vi "RYB_labview_ardunio.vi"() -> ()   [LabVIEW 2013]
uses:
  D:/Program Files (x86)/National Instruments/LabVIEW 2013/examples/Instrument IO/Serial/support/Serial - Settings.ctl
  <vilib>/Instr/_visa.llb/VISA Configure Serial Port (Instr).vi
panel:
  out "B":dbl
  out "Y":dbl
  out "R":dbl
  in  "Boolean 5":bool
  out "B PHASE":bool
  out "Y PHASE":bool
  out "R PHASE":bool
  in  "stop":bool
  out "Input Data":i32(graph)
  out "FSR1":string
  out "Input buffer":string
  in  "byte count":u32
  in  "Serial Settings":T1={"baud rate"=9600, "data bits"=8, "parity"=enum."None", "stop bits"=10, "flow control"=0} {"flow control" items=["None"=0, "XON/XOFF"=1, "RTS/CTS"=2, "DTR/DSR"=4]; "stop bits" items=["1.0"=10, "1.5"=15, "2.0"=20]; "data bits" min=5 max=8 step=1; "baud rate" items=["75"=75, "110"=110, "134"=134, "150"=150, "300"=300, "600"=600, "1200"=1200, "1800"=1800, "2400"=2400, "4800"=4800, "7200"=7200, "9600"=9600, "14400"=14400, "19200"=19200, "28800"=28800, "38400"=38400, "56000"=56000, "57600"=57600, "115200"=115200, "128000"=128000, "230400"=230400]}
  in  "VISA resource name":refnum<visa-resource-name>
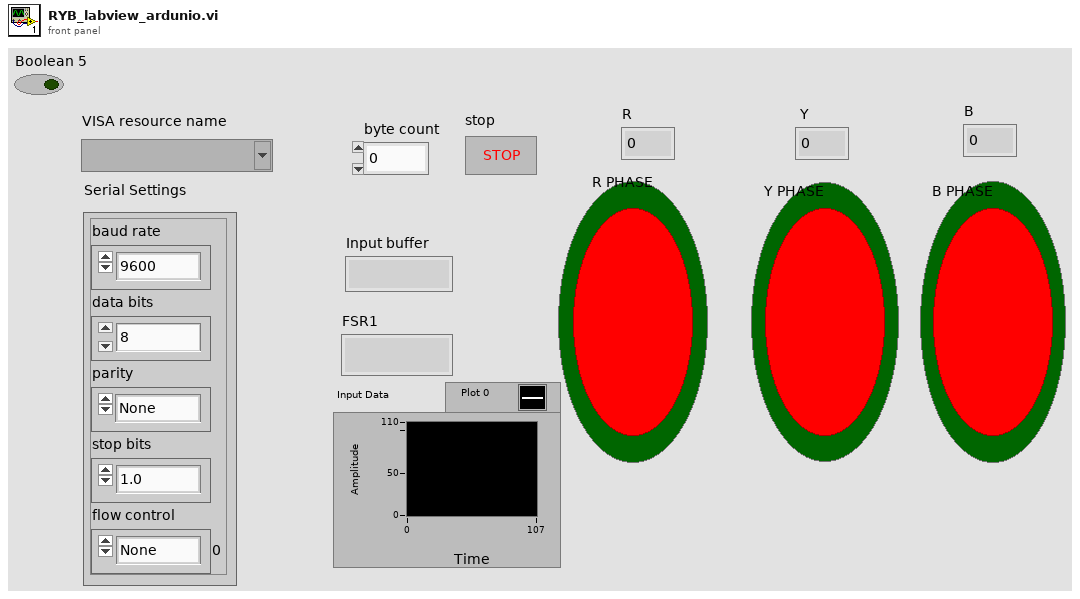
[diagram p1: front panel]
types:
  T1 = typedef "Serial - Settings.ctl" = cluster{"baud rate":u32, "data bits":u16, "parity":enum16{"None", "Odd", "Even", "Mark", "Space"}, "stop bits":u16, "flow control":u16}
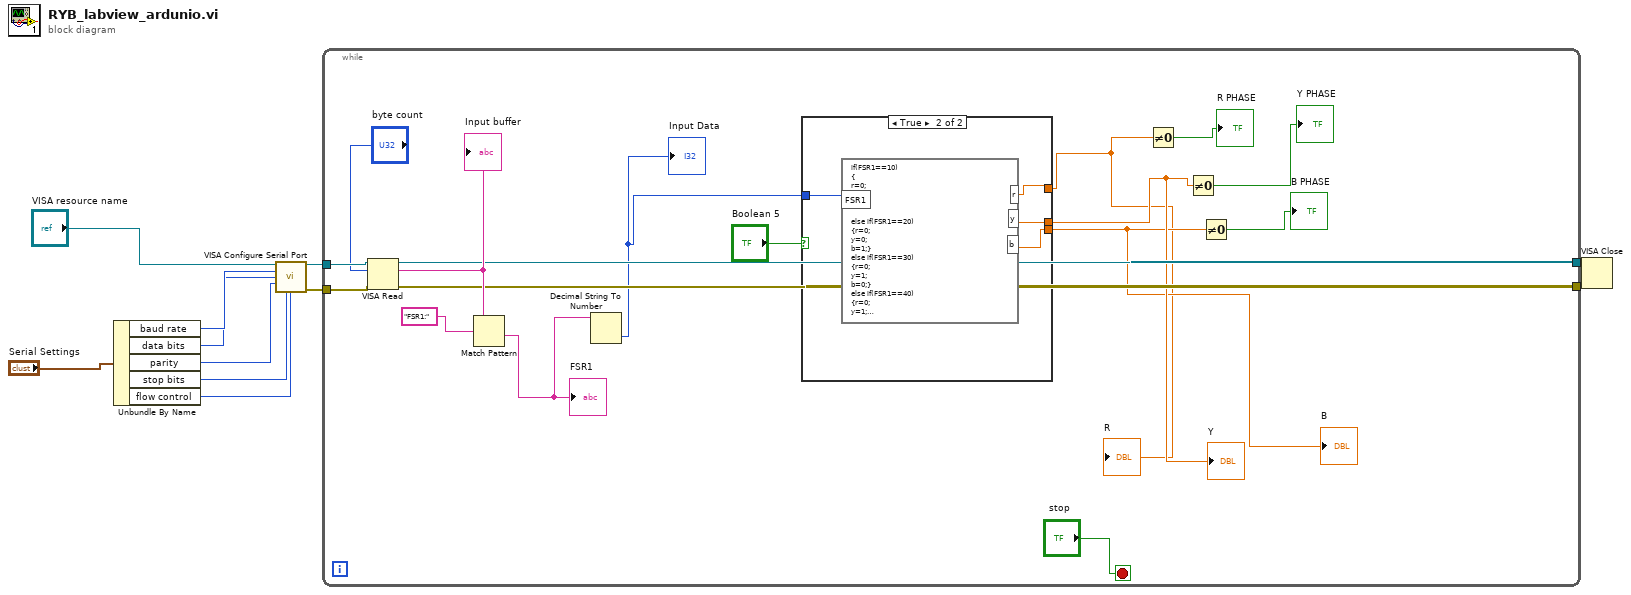
[diagram p0: block diagram]
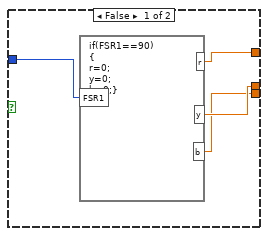
[diagram p2: hidden frame]
diagram:
  n1 = Unbundle By Name("Serial Settings") -> ("baud rate"=w9:u32, "data bits"=w8:u16, "parity"=w7:enum16{"None", "Odd", "Even", "Mark", "Space"}, "stop bits"=w6:u16, "flow control"=w5:u16)
  n2 = call-poly "VISA Configure Serial Port"("VISA resource name"="VISA resource name", "baud rate (9600)"=w9, "data bits (8)"=w8, "parity (0:none)"=w7, "stop bits (10: 1 bit)"=w6, "flow control (0:none)"=w5) -> ("VISA resource name out"=w4:refnum<visa-resource-name>, "error out"=w3:errorcluster)  [unwired: 8 in]
  n3 = while {
    tunnel: w4 -> [w28]
    tunnel: w3 -> [w27]
    tunnel: [w23] -> w2
    tunnel: [w22] -> w1
    stop <- "stop" stop-if-true
    n4 = VISA Read(VISA resource name=w28, byte count="byte count", error in (no error)=w27) -> (VISA resource name out=w22:refnum<visa-resource-name>, read buffer=w25:string, error out=w23:errorcluster)  [unwired: 1 out]
    "Input buffer" <- w25
    n5 = Match Pattern(string=w25, regular expression="FSR1:") -> (after substring=w20:string)  [unwired: 1 in, 3 out]
    "FSR1" <- w20
    n6 = Decimal String To Number(string=w20) -> (number=w17:i32)  [unwired: 2 in, 1 out]
    "Input Data" <- w17
    n7 = case shown="True" "Boolean 5" {
      tunnel: w17 -> [w32 w36]
      tunnel: [w30 w35] -> w15
      tunnel: [w29 w34] -> w14
      tunnel: [w31 w33] -> w12
      frame False {
        n8 = formula code="if(FSR1==90)\n{\nr=0;\ny=0;\nb=0;}"("FSR1"=w32) -> ("r"=w31:dbl, "y"=w30:dbl, "b"=w29:dbl)
      }
      frame True {
        n9 = formula code="if(FSR1==10)\n{\nr=0;\ny=0;\nb=0;}\n\nelse if(FSR1==20)\n{r=0;\ny=0;\nb=1;}\nelse if(FSR1==30)\n{r=0;\ny=1;\nb=0;}\nelse if(FSR1==40)\n{r=0;\ny=1;\nb=1;}\nelse if(FSR1==50)\n{r=1;\ny=0;\nb=0;}\nelse if(FSR1==60)\n{r=1;\ny=0;\nb=1;}\nelse if(FSR1==70)\n{r=1;\ny=1;\nb=0;}\nelse if(FSR1==80)\n{r=1;\ny=1;\nb=1;}"("FSR1"=w36) -> ("r"=w33:dbl, "y"=w35:dbl, "b"=w34:dbl)
      }
    }
    "R" <- w12
    "Y" <- w15
    "B" <- w14
    n10 = Not Equal To 0?(x=w12) -> (x != 0?=→"R PHASE":bool)
    n11 = Not Equal To 0?(x=w15) -> (x != 0?=→"Y PHASE":bool)
    n12 = Not Equal To 0?(x=w14) -> (x != 0?=→"B PHASE":bool)
  }
  n13 = VISA Close(VISA resource name=w1, error in (no error)=w2) -> ()  [unwired: 1 out]
